vi "Acquire.vi"(8 "error in":errorcluster, 10 "configuration":T1, 11 "session":T2) -> (0 "error out":errorcluster, 2 "Digital waveform":u32[][](array[numeric]), 3 "No of Samples per channel":u32)   [LabVIEW 2021, in "dcvmDPI_AD7606B_serverImpl.lvlib"]
uses:
  dcvmDPI_AD7606B_serverImpl.lvlib
  controls/session.ctl
  controls/configuration.ctl
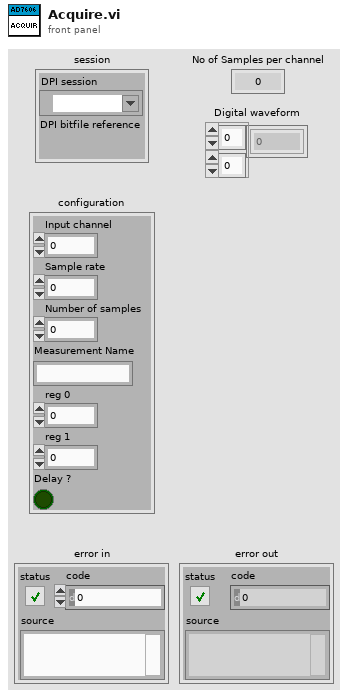
[diagram p1: front panel]
types:
  T1 = typedef "dcvmDPI_AD7606B_serverImpl.lvlib/configuration.ctl" = cluster{"Input channel":i32, "Sample rate":dbl, "Number of samples":u32, "Measurement Name":string, "reg 0":i32, "reg 1":i32, "Delay ?":bool}
  T2 = typedef "dcvmDPI_AD7606B_serverImpl.lvlib/session.ctl" = cluster{"DPI session":refnum<k15>, "DPI bitfile reference":refnum<k20>}
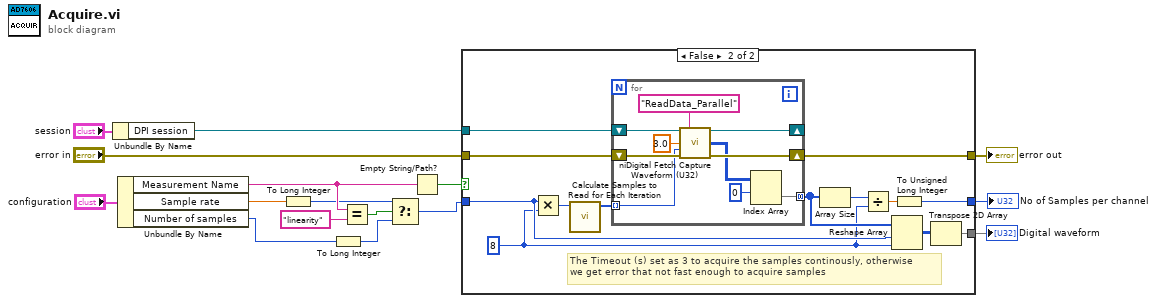
[diagram p0: block diagram]
diagram:
  n1 = Unbundle By Name("session") -> ("DPI session"=w12:refnum<k15>)
  n2 = Unbundle By Name("configuration") -> ("Measurement Name"=w8:string, "Sample rate"=w3:dbl, "Number of samples"=w5:u32)
  n3 = To Long Integer(number=w3) -> (32bit integer=w2:i32)
  n4 = To Long Integer(number=w5) -> (32bit integer=w4:i32)
  n5 = Equal?(x=w8, y="linearity") -> (x = y?=w6:bool)
  n6 = Select(t=w2, s=w6, f=w4) -> (s? t:f=w1:i32)
  n7 = Empty String/Path?(string/path=w8) -> (empty?=w10:bool)
  n8 = case shown="False" w10 {
    tunnel: [w17 w30] -> w16
    tunnel: "error in" -> [w17 w29]
    tunnel: w12 -> [_ w28]
    tunnel: w1 -> [_ w23]
    tunnel: [_ w26] -> w11
    tunnel: [_ w18] -> w9
    frame True {
    }
    frame False {
      w20 = 8 ("x")
      # "The Timeout (s) set as 3 to acquire the samples continously, otherwise \nwe get error that not fast enough to acquire samples"
      n9 = Multiply(x=w23, y=w20) -> (x*y=w24:i32)
      n10 = call "Calculate Samples to Read for Each Iteration.vi"("total samples to read"=w24) -> ("samples to read"=w25:i32[])  [unwired: 10 in]
      n11 = for {
        tunnel: w25 -> [w31] mode=indexing
        shift-right: [w35] -> _
        shift-left: w28 -> [w40]
        shift-right: [w34] -> w30
        shift-left: w29 -> [w39]
        tunnel: [w36] -> w22 mode=concatenating
        n12 = call <instrlib>:"niDigital Fetch Capture Waveform (U32).vi"("instrument handle"=w40, "waveform name"="ReadData_Parallel", "timeout (s)"=3.0, "samples to read"=w31, "error in"=w39) -> ("instrument handle out"=w35:refnum<k15>, "data"=w32:u32[][], "error out"=w34:errorcluster)  [unwired: 8 in]
        n13 = Index Array(array=w32, index (row)=0) -> (element=w36:u32[])  [unwired: 1 in]
      }
      n14 = Array Size(array=w22) -> (size(s)=w21:i32)
      n15 = Divide(x=w21, y=w20) -> (x/y=w19:dbl)
      n16 = Reshape Array(w22, w23, w20) -> (w27:u32[][])
      n17 = To Unsigned Long Integer(number=w19) -> (unsigned 32bit integer=w18:u32)
      n18 = Transpose 2D Array(2D array=w27) -> (transposed array=w26:u32[][])
    }
  }
  "error out" <- w16
  "Digital waveform" <- w11
  "No of Samples per channel" <- w9
